vi "TRTDM Analyze Temp Measurements.vi"(0 "Temperature Waveforms In":waveform(dbl)[](array[waveform]), 11 "error in (no error)":errorcluster) -> (4 "Measure Settings":T1 {"Average Temperature (K)" format="%.2p"; "Average Temperature (deg C)" format="%.2p"}, 15 "error out":errorcluster)   [LabVIEW 2021, in "DAQ_Temperature RTD Measurement.lvlib"]
doc: "Analyzes the temperature RTD waveforms data obtained from analog input temperature measurements to derive required average temperature measurements"
uses:
  DAQ_Temperature RTD Measurement.lvlib
  Typedefs/Temperature RTD Measurements.ctl
  <vilib>/Analysis/baseanly.llb/Mean (DBL).vi
  <vilib>/Analysis/NI_AALBase.lvlib
panel:
  # "Inputs"
  # "Outputs"
  # "Overview:\nThis VI does post processing on obtained temperature waveforms from analog input temperature measurements to give the requiredTemperature Measurements output\n\nInstructions:\n1. Input the captured temperature waveforms to the input controls\n2. Observe the analyzed Temperature measurements output"
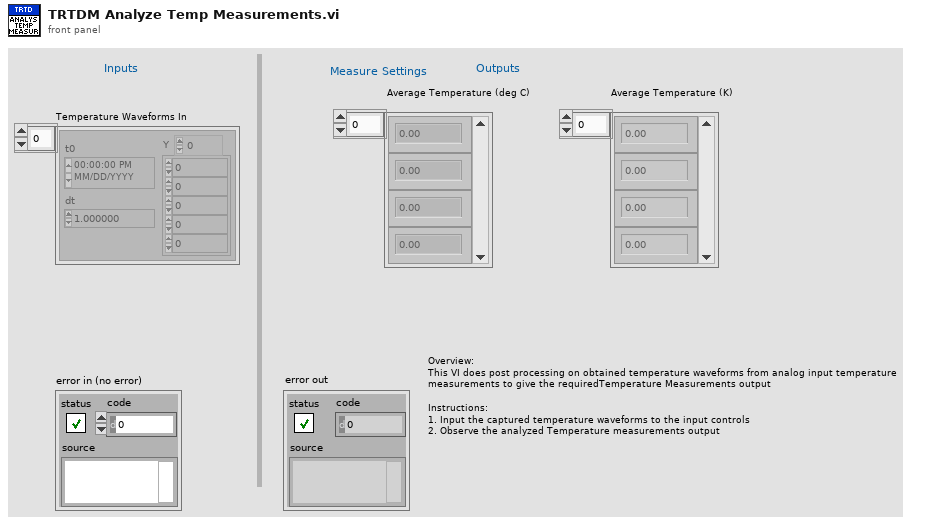
[diagram p1: front panel]
types:
  T1 = typedef "DAQ_Temperature RTD Measurement.lvlib/Temperature RTD Measurements.ctl" = cluster{"Average Temperature (deg C)":dbl[], "Average Temperature (K)":dbl[]}
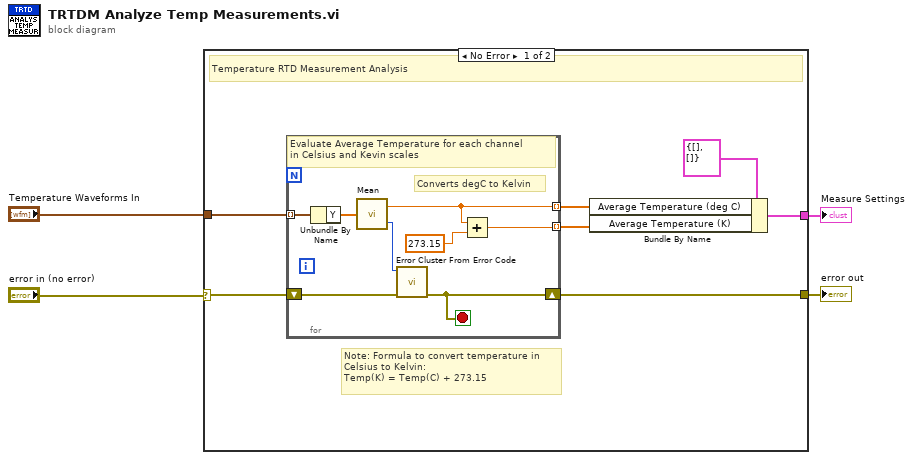
[diagram p0: block diagram]
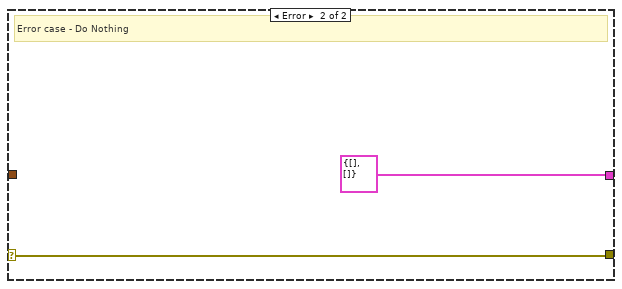
[diagram p2: hidden frame]
diagram:
  n1 = case shown="No Error" "error in (no error)" {
    selector: "error in (no error)" -> [w9 w21]
    tunnel: "Temperature Waveforms In" -> [w7 _]
    tunnel: [w10 T1 {"Average Temperature (deg C)"=[], "Average Temperature (K)"=[]} ("Measure Settings")] -> w1
    tunnel: [w8 w21] -> w2
    frame No Error {
      # "Note: Formula to convert temperature in\nCelsius to Kelvin:\nTemp(K) = Temp(C) + 273.15"
      # "Temperature RTD Measurement Analysis"
      n2 = for {
        shift-right: [w13] -> w8
        shift-left: w9 -> [w14]
        tunnel: w7 -> [w19] mode=indexing
        tunnel: [w16] -> w6 mode=indexing
        tunnel: [w15] -> w5 mode=indexing
        stop <- w13 stop-if-true
        # "Converts degC to Kelvin"
        # "Evaluate Average Temperature for each channel\nin Celsius and Kevin scales"
        n3 = Unbundle By Name(w19) -> ("Y"=w18:dbl[])
        n4 = call-poly <vilib>:"Mean.vi"("X"=w18) -> ("mean"=w16:dbl, "error"=w12:i32)
        n5 = call <vilib>:"Error Cluster From Error Code.vi"("error in (no error)"=w14, "error code (0)"=w12) -> ("error out"=w13:errorcluster)  [unwired: 7 in]
        n6 = Add(x=w16, y=273.15) -> (x+y=w15:dbl)
      }
      n7 = Bundle By Name(cluster=T1 {"Average Temperature (deg C)"=[], "Average Temperature (K)"=[]} ("Measure Settings"), "Average Temperature (deg C)"=w6, "Average Temperature (K)"=w5) -> (w10:T1)
    }
    frame Error {
      # "Error case - Do Nothing"
    }
  }
  "error out" <- w2
  "Measure Settings" <- w1
